vi "control2.vi"   [LabVIEW 2020]
uses:
  enum.ctl
  G_Estados_Elevador.vi
  G_Estados_Desmenuzadora.vi
  G_Posiciones_Variables.vi
  G_PalaDeGrua.vi
  G_Estados_Rotativa.vi
  G_Horno.vi
  G_Enfriamiento.vi
types:
  T1 = cluster{"Masa tolva":bool, "Rodillo 1":bool, "Rodillo 2":bool, "Galletas":bool, "Banda 1":bool}
  T2 = typedef "enum.ctl" = enum16{"pala grua", "desmezuradora", "elevador", "rotativa", "horneado", "enfriamiento"}
  T3 = cluster{"Desmenuzadora (x)":i32, "Desmenuzadora (y)":i32, "Aspa (x)":i32, "Aspa (y)":i32, "Masa elevador (x)":i32, "Masa elevador (y) ":i32, "Galletas Molde (x)":i32, "Galletas Molde (y)":i32, "Galletas Horno (x) ":i32, "Galletas Horno (y) ":i32, "Galletas Enfria (x) ":i32, "Galletas Enfria (y) ":i32}
  T4 = cluster{"Llama horno":bool, "Termometro":dbl, "Galletas Horno":bool, "Banda 2":bool, "Banda 3":bool}
  T5 = cluster{"Banda 4":bool, "Banda 5":bool, "Banda 6":bool, "Galletas Enfria":bool}
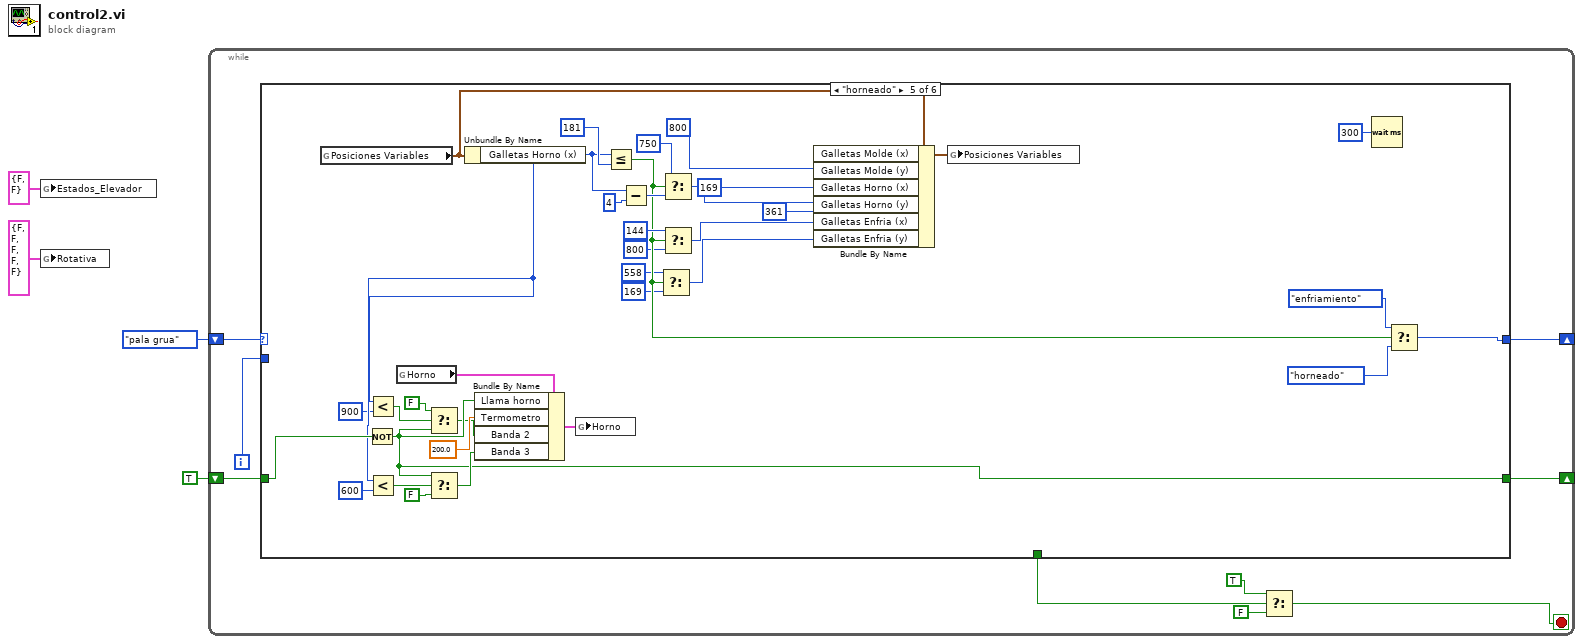
[diagram p0: block diagram]
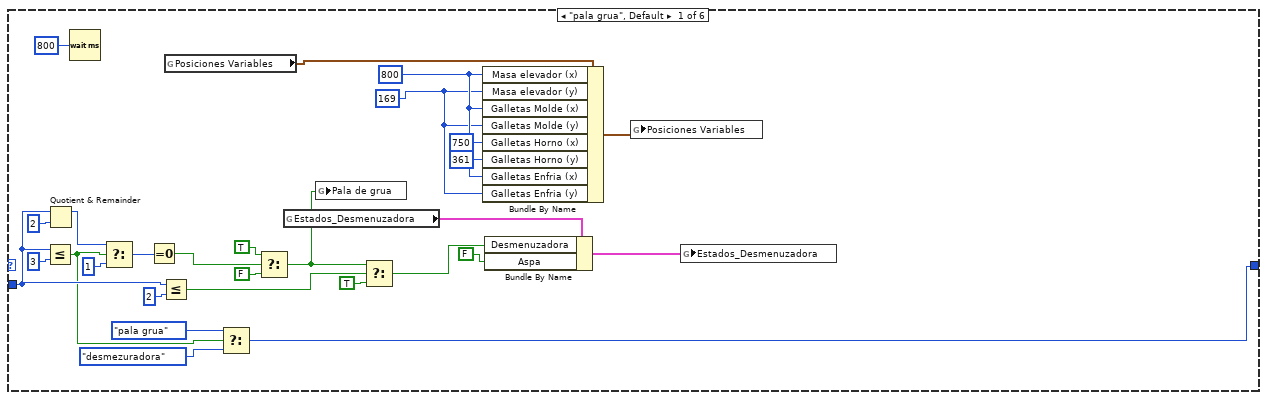
[diagram p2: hidden frame]
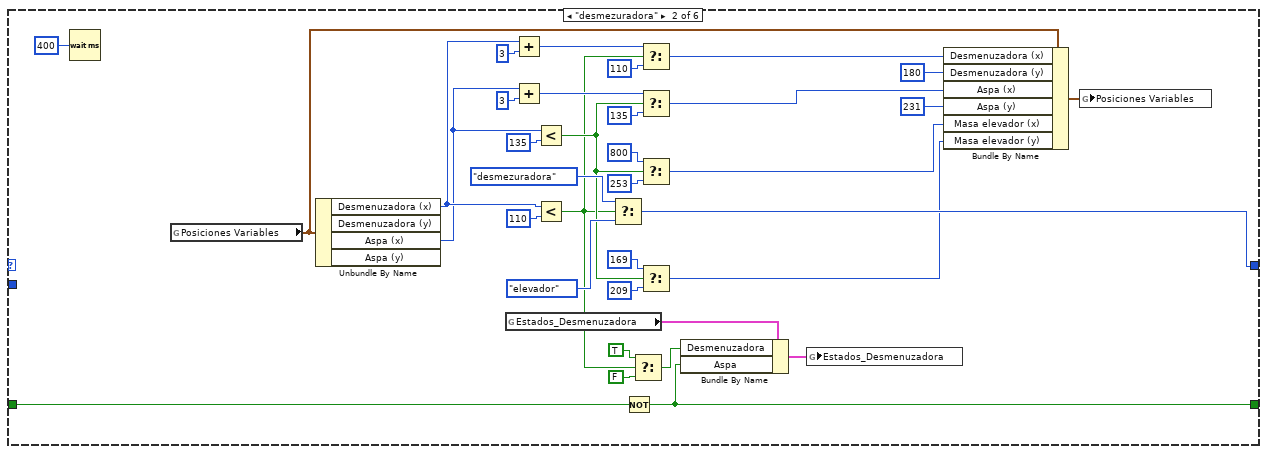
[diagram p3: hidden frame]
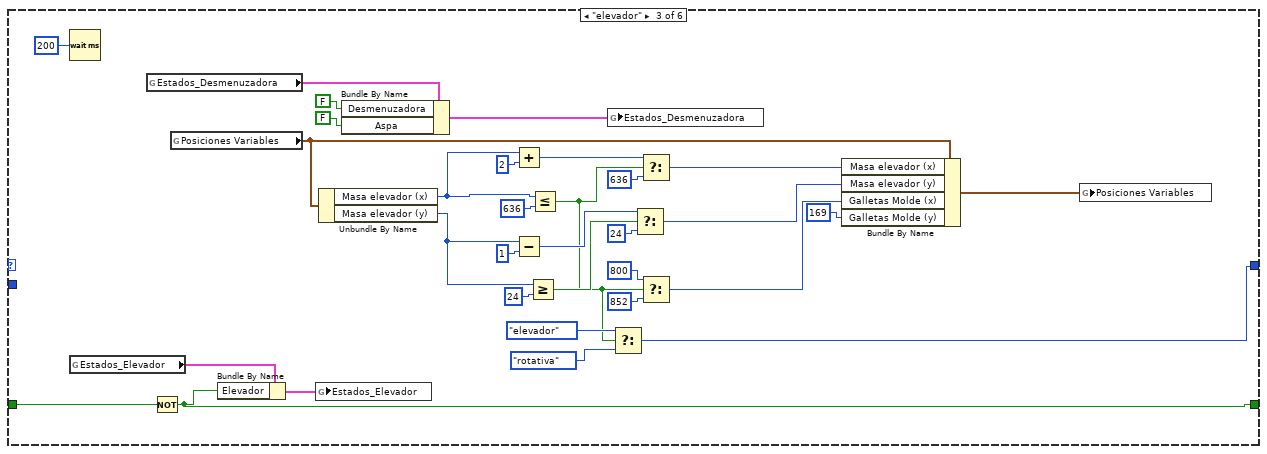
[diagram p4: hidden frame]
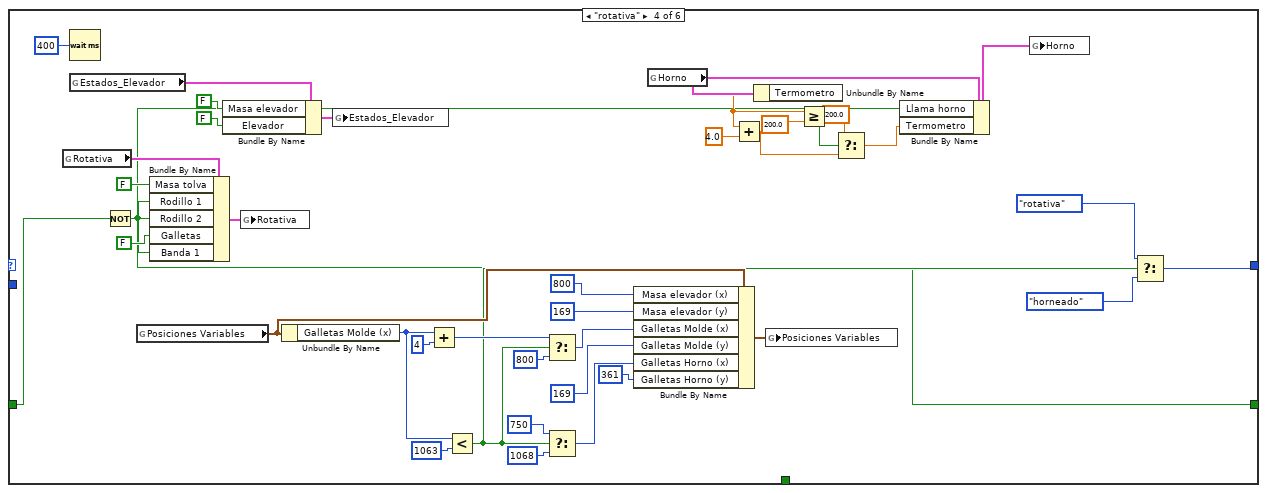
[diagram p5: hidden frame]
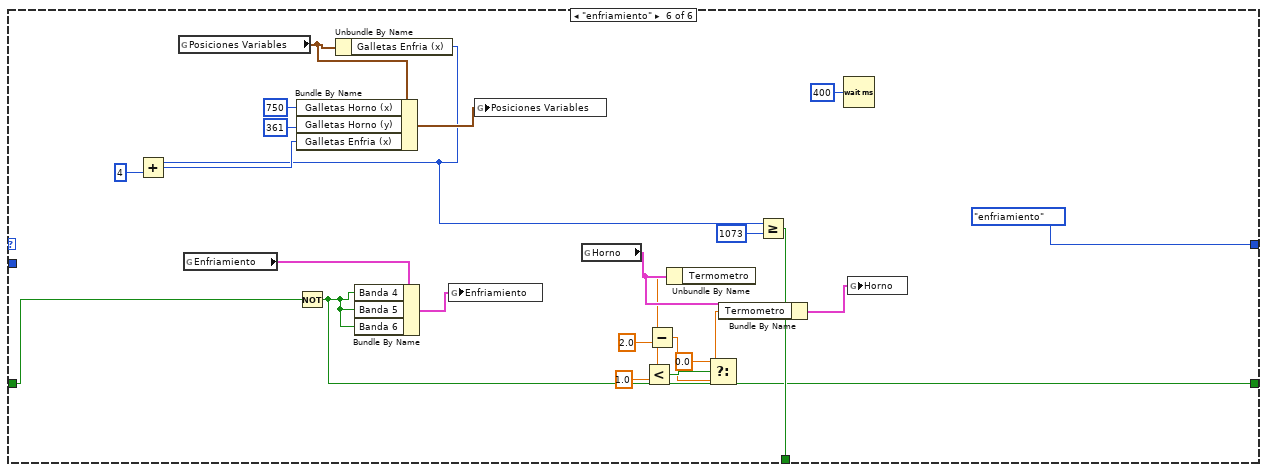
[diagram p6: hidden frame]
diagram:
  n1 = global write "G_Estados_Elevador.vi" "Estados_Elevador"(cluster{"Masa elevador":bool, "Elevador":bool} {"Masa elevador"=FALSE, "Elevador"=FALSE} ("Estados_Elevador")) -> ()
  n2 = global write "G_Estados_Rotativa.vi" "Rotativa"(T1 {"Masa tolva"=FALSE, "Rodillo 1"=FALSE, "Rodillo 2"=FALSE, "Galletas"=FALSE, "Banda 1"=FALSE} ("Rotativa")) -> ()
  n3 = while {
    shift-right: [w11] -> _
    shift-left: enum."pala grua" -> [w13]
    shift-right: [w9] -> _
    shift-left: TRUE -> [w10]
    i -> [w12]
    stop <- w6 stop-if-true
    n4 = case shown="\"horneado\"" w13 {
      tunnel: w12 -> [w28 _ _ _ _ _]
      tunnel: [w20 w56 w84 w119 w175 enum."enfriamiento"] -> w11
      tunnel: w10 -> [_ w55 w101 w138 w170 w195]
      tunnel: [_ w54 w100 w109 w150 w183] -> w9
      tunnel: [_ _ _ _ _ w198] -> w5
      frame "pala grua", Default {
        w14 = 169 ("Masa elevador (y)")
        w15 = 800 ("Masa elevador (x)")
        n5 = Less Or Equal?(x=w28, y=3) -> (x <= y?=w23:bool)
        n6 = Quotient & Remainder(x=w28, y=2) -> (x-y*floor(x/y)=w33:i32)  [unwired: 1 out]
        n7 = Wait (ms)(milliseconds to wait=u32 800) -> ()  [unwired: 1 out]
        n8 = Select(t=w33, s=w23, f=1) -> (s? t:f=w34:i32)
        n9 = Equal To 0?(x=w34) -> (x = 0?=w38:bool)
        n10 = Less Or Equal?(x=w28, y=2) -> (x <= y?=w31:bool)
        n11 = global read "G_Posiciones_Variables.vi" "Posiciones Variables"() -> (w19:T3)
        n12 = Select(t=enum."pala grua", s=w23, f=enum."desmezuradora") -> (s? t:f=w20:T2)
        n13 = Select(t=TRUE, s=w38, f=FALSE) -> (s? t:f=w29:bool)
        n14 = global read "G_Estados_Desmenuzadora.vi" "Estados_Desmenuzadora"() -> (w26:cluster{"Desmenuzadora":bool, "Aspa":bool})
        n15 = global write "G_PalaDeGrua.vi" "Pala de grua"(w29) -> ()
        n16 = Select(t=w29, s=w31, f=TRUE) -> (s? t:f=w25:bool)
        n17 = Bundle By Name(cluster=w19, "Masa elevador (x)"=w15, "Masa elevador (y)"=w14, "Galletas Molde (x)"=w15, "Galletas Molde (y)"=w14, "Galletas Horno (x)"=750, "Galletas Horno (y)"=361, "Galletas Enfria (x)"=w15, "Galletas Enfria (y)"=w14) -> (w18:T3)
        n18 = Bundle By Name(cluster=w26, "Desmenuzadora"=w25, "Aspa"=FALSE) -> (w27:cluster{"Desmenuzadora":bool, "Aspa":bool})
        n19 = global write "G_Posiciones_Variables.vi" "Posiciones Variables"(w18) -> ()
        n20 = global write "G_Estados_Desmenuzadora.vi" "Estados_Desmenuzadora"(w27) -> ()
      }
      frame "desmezuradora" {
        n21 = Wait (ms)(milliseconds to wait=u32 400) -> ()  [unwired: 1 out]
        n22 = global read "G_Posiciones_Variables.vi" "Posiciones Variables"() -> (w74:T3)
        n23 = Unbundle By Name(w74) -> ("Desmenuzadora (x)"=w72:i32, "Aspa (x)"=w62:i32)  [unwired: 2 out]
        n24 = global read "G_Estados_Desmenuzadora.vi" "Estados_Desmenuzadora"() -> (w59:cluster{"Desmenuzadora":bool, "Aspa":bool})
        n25 = Add(x=w72, y=3) -> (x+y=w70:i32)
        n26 = Add(x=w62, y=3) -> (x+y=w50:i32)
        n27 = Less?(x=w62, y=135) -> (x < y?=w46:bool)
        n28 = Less?(x=w72, y=110) -> (x < y?=w45:bool)
        n29 = Select(t=enum."desmezuradora", s=w45, f=enum."elevador") -> (s? t:f=w56:T2)
        n30 = Not(x=w55) -> (.not. x?=w54:bool)
        n31 = Select(t=TRUE ("Desmenuzadora"), s=w45, f=FALSE) -> (s? t:f=w42:bool)
        n32 = Select(t=w70, s=w45, f=110) -> (s? t:f=w68:i32)
        n33 = Select(t=w50, s=w46, f=135) -> (s? t:f=w64:i32)
        n34 = Select(t=i64 800, s=w46, f=i64 253) -> (s? t:f=w53:i64)
        n35 = Select(t=169, s=w46, f=209) -> (s? t:f=w47:i32)
        n36 = Bundle By Name(cluster=w59, "Desmenuzadora"=w42, "Aspa"=w54) -> (w60:cluster{"Desmenuzadora":bool, "Aspa":bool})
        n37 = global write "G_Estados_Desmenuzadora.vi" "Estados_Desmenuzadora"(w60) -> ()
        n38 = Bundle By Name(cluster=w74, "Desmenuzadora (x)"=w68, "Desmenuzadora (y)"=180, "Aspa (x)"=w64, "Aspa (y)"=231, "Masa elevador (x)"=w53, "Masa elevador (y)"=w47) -> (w61:T3)
        n39 = global write "G_Posiciones_Variables.vi" "Posiciones Variables"(w61) -> ()
      }
      frame "elevador" {
        n40 = Wait (ms)(milliseconds to wait=u32 200) -> ()  [unwired: 1 out]
        n41 = global read "G_Estados_Elevador.vi" "Estados_Elevador"() -> (w103:cluster{"Masa elevador":bool, "Elevador":bool})
        n42 = global read "G_Estados_Desmenuzadora.vi" "Estados_Desmenuzadora"() -> (w107:cluster{"Desmenuzadora":bool, "Aspa":bool})
        n43 = Not(x=w101) -> (.not. x?=w100:bool)
        n44 = global read "G_Posiciones_Variables.vi" "Posiciones Variables"() -> (w98:T3)
        n45 = Bundle By Name(cluster=w103, "Elevador"=w100) -> (w102:cluster{"Masa elevador":bool, "Elevador":bool})
        n46 = global write "G_Estados_Elevador.vi" "Estados_Elevador"(w102) -> ()
        n47 = Unbundle By Name(w98) -> ("Masa elevador (x)"=w90:i32, "Masa elevador (y)"=w95:i32)
        n48 = Bundle By Name(cluster=w107, "Desmenuzadora"=FALSE, "Aspa"=FALSE) -> (w108:cluster{"Desmenuzadora":bool, "Aspa":bool})
        n49 = Add(x=w90, y=2) -> (x+y=w88:i32)
        n50 = Subtract(x=w95, y=1) -> (x-y=w93:i32)
        n51 = Greater Or Equal?(x=w95, y=24) -> (x >= y?=w79:bool)
        n52 = Less Or Equal?(x=w90, y=636) -> (x <= y?=w77:bool)
        n53 = global write "G_Estados_Desmenuzadora.vi" "Estados_Desmenuzadora"(w108) -> ()
        n54 = Select(t=enum."elevador", s=w77, f=enum."rotativa") -> (s? t:f=w84:T2)
        n55 = Select(t=w93, s=w79, f=24) -> (s? t:f=w91:i32)
        n56 = Select(t=w88, s=w77, f=636) -> (s? t:f=w83:i32)
        n57 = Select(t=800, s=w77, f=852 ("Galletas Molde (x)")) -> (s? t:f=w80:i32)
        n58 = Bundle By Name(cluster=w98, "Masa elevador (x)"=w83, "Masa elevador (y)"=w91, "Galletas Molde (x)"=w80, "Galletas Molde (y)"=169) -> (w97:T3)
        n59 = global write "G_Posiciones_Variables.vi" "Posiciones Variables"(w97) -> ()
      }
      frame "rotativa" {
        n60 = global read "G_Estados_Rotativa.vi" "Rotativa"() -> (w142:T1)
        n61 = Wait (ms)(milliseconds to wait=u32 400) -> ()  [unwired: 1 out]
        n62 = global read "G_Estados_Elevador.vi" "Estados_Elevador"() -> (w147:cluster{"Masa elevador":bool, "Elevador":bool})
        n63 = Not(x=w138) -> (.not. x?=w109:bool)
        n64 = global read "G_Posiciones_Variables.vi" "Posiciones Variables"() -> (w134:T3)
        n65 = Bundle By Name(cluster=w142, "Masa tolva"=FALSE, "Rodillo 1"=w109, "Rodillo 2"=w109, "Galletas"=FALSE, "Banda 1"=w109) -> (w143:T1)
        n66 = Bundle By Name(cluster=w147, "Masa elevador"=FALSE, "Elevador"=FALSE) -> (w146:cluster{"Masa elevador":bool, "Elevador":bool})
        n67 = global write "G_Estados_Rotativa.vi" "Rotativa"(w143) -> ()
        n68 = Unbundle By Name(w134) -> ("Galletas Molde (x)"=w132:i32)
        n69 = global write "G_Estados_Elevador.vi" "Estados_Elevador"(w146) -> ()
        n70 = Add(x=w132, y=4) -> (x+y=w130:i32)
        n71 = Less?(x=w132, y=1063) -> (x < y?=w122:bool)
        n72 = Select(t=w130, s=w122, f=800) -> (s? t:f=w128:i32)
        n73 = Select(t=750, s=w122, f=1068) -> (s? t:f=w123:i32)
        n74 = Bundle By Name(cluster=w134, "Masa elevador (x)"=800, "Masa elevador (y)"=169, "Galletas Molde (x)"=w128, "Galletas Molde (y)"=169, "Galletas Horno (x)"=w123, "Galletas Horno (y)"=361) -> (w137:T3)
        n75 = global read "G_Horno.vi" "Horno"() -> (w117:T4)
        n76 = Unbundle By Name(w117) -> ("Termometro"=w115:dbl)
        n77 = Add(x=w115, y=4.0) -> (x+y=w111:dbl)
        n78 = global write "G_Posiciones_Variables.vi" "Posiciones Variables"(w137) -> ()
        n79 = Greater Or Equal?(x=w115, y=200.0) -> (x >= y?=w113:bool)
        n80 = Select(t=200.0, s=w113, f=w111) -> (s? t:f=w110:dbl)
        n81 = Bundle By Name(cluster=w117, "Llama horno"=w109, "Termometro"=w110) -> (w116:T4)
        n82 = global write "G_Horno.vi" "Horno"(w116) -> ()
        n83 = Select(t=enum."rotativa", s=w122, f=enum."horneado") -> (s? t:f=w119:T2)
      }
      frame "horneado" {
        n84 = global read "G_Posiciones_Variables.vi" "Posiciones Variables"() -> (w179:T3)
        n85 = Not(x=w170) -> (.not. x?=w150:bool)
        n86 = global read "G_Horno.vi" "Horno"() -> (w172:T4)
        n87 = Unbundle By Name(w179) -> ("Galletas Horno (x)"=w154:i32)
        n88 = Less?(x=w154, y=900) -> (x < y?=w152:bool)
        n89 = Less?(x=w154, y=600) -> (x < y?=w168:bool)
        n90 = Select(t=FALSE, s=w152, f=w150) -> (s? t:f=w149:bool)
        n91 = Select(t=w150, s=w168, f=FALSE) -> (s? t:f=w165:bool)
        n92 = Bundle By Name(cluster=w172, "Llama horno"=w150, "Termometro"=200.0, "Banda 2"=w149, "Banda 3"=w165) -> (w171:T4)
        n93 = global write "G_Horno.vi" "Horno"(w171) -> ()
        n94 = Less Or Equal?(x=w154, y=181) -> (x <= y?=w160:bool)
        n95 = Subtract(x=w154, y=4) -> (x-y=w163:i32)
        n96 = Select(t=558, s=w160, f=169) -> (s? t:f=w156:i32)
        n97 = Select(t=750, s=w160, f=w163) -> (s? t:f=w176:i32)
        n98 = Select(t=144, s=w160, f=800) -> (s? t:f=w162:i32)
        n99 = Bundle By Name(cluster=w179, "Galletas Molde (x)"=800, "Galletas Molde (y)"=169, "Galletas Horno (x)"=w176, "Galletas Horno (y)"=361, "Galletas Enfria (x)"=w162, "Galletas Enfria (y)"=w156) -> (w182:T3)
        n100 = global write "G_Posiciones_Variables.vi" "Posiciones Variables"(w182) -> ()
        n101 = Wait (ms)(milliseconds to wait=u32 300) -> ()  [unwired: 1 out]
        n102 = Select(t=enum."enfriamiento", s=w160, f=enum."horneado") -> (s? t:f=w175:T2)
      }
      frame "enfriamiento" {
        n103 = global read "G_Posiciones_Variables.vi" "Posiciones Variables"() -> (w206:T3)
        n104 = global read "G_Enfriamiento.vi" "Enfriamiento"() -> (w194:T5)
        n105 = Not(x=w195) -> (.not. x?=w183:bool)
        n106 = Unbundle By Name(w206) -> ("Galletas Enfria (x)"=w200:i32)
        n107 = Add(x=w200, y=4) -> (x+y=w201:i32)
        n108 = Bundle By Name(cluster=w206, "Galletas Horno (x)"=750, "Galletas Horno (y)"=361, "Galletas Enfria (x)"=w201) -> (w205:T3)
        n109 = Bundle By Name(cluster=w194, "Banda 4"=w183, "Banda 5"=w183, "Banda 6"=w183) -> (w193:T5)
        n110 = global write "G_Enfriamiento.vi" "Enfriamiento"(w193) -> ()
        n111 = global write "G_Posiciones_Variables.vi" "Posiciones Variables"(w205) -> ()
        n112 = global read "G_Horno.vi" "Horno"() -> (w191:T4)
        n113 = Unbundle By Name(w191) -> ("Termometro"=w188:dbl)
        n114 = Less?(x=w188, y=1.0) -> (x < y?=w186:bool)
        n115 = Subtract(x=w188, y=2.0) -> (x-y=w184:dbl)
        n116 = Select(t=0.0, s=w186, f=w184) -> (s? t:f=w189:dbl)
        n117 = Bundle By Name(cluster=w191, "Termometro"=w189) -> (w192:T4)
        n118 = Greater Or Equal?(x=w200, y=1073) -> (x >= y?=w198:bool)
        n119 = Wait (ms)(milliseconds to wait=u32 400) -> ()  [unwired: 1 out]
        n120 = global write "G_Horno.vi" "Horno"(w192) -> ()
      }
    }
    n121 = Select(t=TRUE, s=w5, f=FALSE) -> (s? t:f=w6:bool)
  }
